vi "Error Cluster From Error Code (nisyscfg).vi"(6 "Details String":string, 8 "error in (no error)":errorcluster, 10 "Error Code (0)":i32, 11 "Details Caption":string) -> (0 "error out":errorcluster)   [LabVIEW 2020, in "nisyscfg.lvlib"]
uses:
  <vilib>/nisyscfg/nisyscfg.lvlib
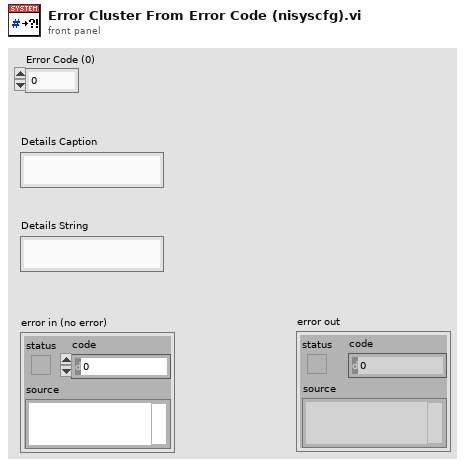
[diagram p1: front panel]
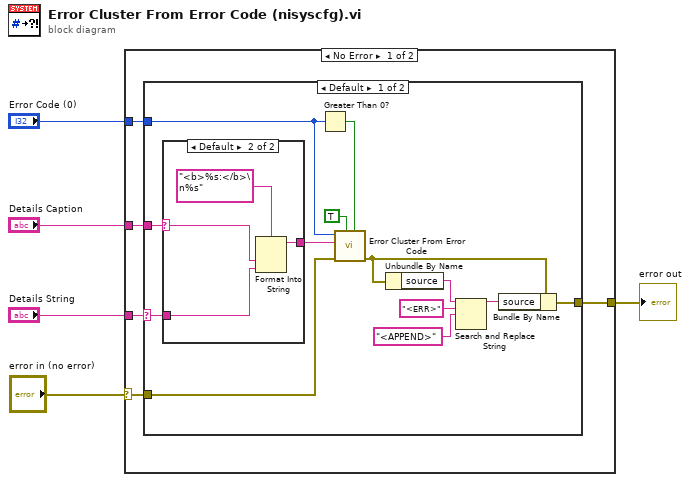
[diagram p0: block diagram]
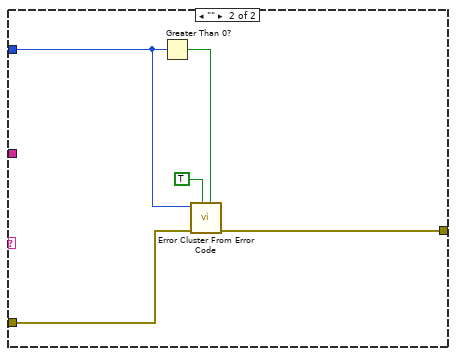
[diagram p3: hidden frame]
diagram:
  n1 = case shown="No Error" "error in (no error)" {
    selector: "error in (no error)" -> [w6 w34]
    tunnel: "Details String" -> [w10 _]
    tunnel: "Error Code (0)" -> [w9 _]
    tunnel: [w8 w34] -> w3
    tunnel: "Details Caption" -> [w7 _]
    frame No Error {
      n2 = case shown="Default" w10 {
        selector: w10 -> [w23 _]
        tunnel: w6 -> [w20 w33]
        tunnel: w9 -> [w12 w30]
        tunnel: [w18 w31] -> w8
        tunnel: w7 -> [w13 _]
        frame Default {
          n3 = case shown="Default" w13 {
            selector: w13 -> [_ w25]
            tunnel: w23 -> [w24 w27]
            tunnel: [w24 w26] -> w21
            frame "" {
            }
            frame Default {
              n4 = Format Into String(format string="<b>%s:</b>\n%s", w25, w27) -> (resulting string=w26:string)  [unwired: 2 in, 1 out]
            }
          }
          n5 = Greater Than 0?(x=w12) -> (x > 0?=w11:bool)
          n6 = call <vilib>:"Error Cluster From Error Code.vi"("is warning? (False)"=w11, "show call chain? (False)"=TRUE, "error in (no error)"=w20, "error message (\"\")"=w21, "error code (0)"=w12) -> ("error out"=w19:errorcluster)  [unwired: 4 out]
          n7 = Unbundle By Name(w19) -> ("source"=w17:string)
          n8 = Search and Replace String(input string=w17, search string="<ERR>", replace string="<APPEND>" ("replace string (\"\")")) -> (result string=w16:string)  [unwired: 5 in, 3 out]
          n9 = Bundle By Name(cluster=w19, "source"=w16) -> (w18:errorcluster)
        }
        frame "" {
          n10 = Greater Than 0?(x=w30) -> (x > 0?=w29:bool)
          n11 = call <vilib>:"Error Cluster From Error Code.vi"("is warning? (False)"=w29, "show call chain? (False)"=TRUE, "error in (no error)"=w33, "error code (0)"=w30) -> ("error out"=w31:errorcluster)  [unwired: 5 out]
        }
      }
    }
    frame Error {
    }
  }
  "error out" <- w3
